vi "5.vi"(8 "error in (no error)":errorcluster) -> (0 "error out":errorcluster, 3 "Voltage":dbl)   [LabVIEW 2015]
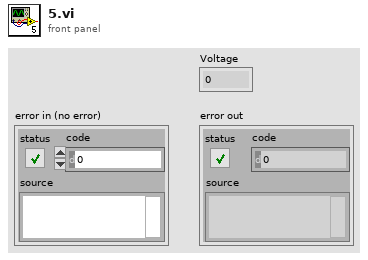
[diagram p1: front panel]
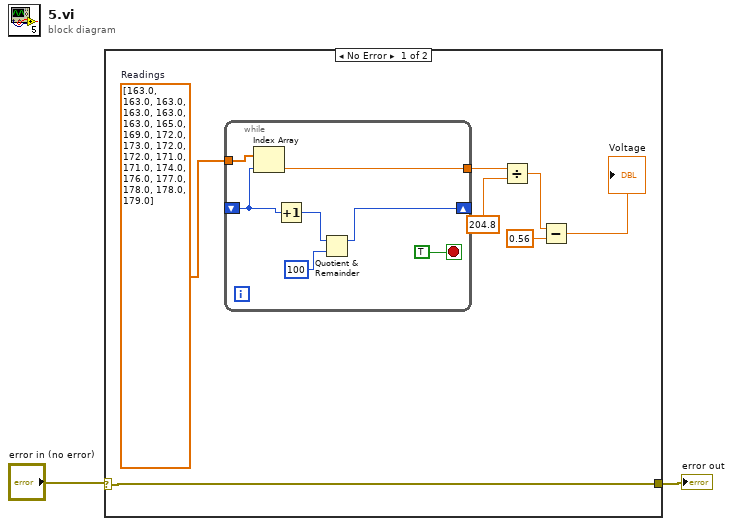
[diagram p0: block diagram]
diagram:
  n1 = case shown="No Error" "error in (no error)" {
    selector: "error in (no error)" -> [w3 w17]
    tunnel: [w3 w17] -> w1
    frame No Error {
      w4 = dbl[] [163.0, 163.0, 163.0, 163.0, 163.0, 163.0, 165.0, 169.0, 172.0, 173.0, 172.0, 172.0, 171.0, 171.0, 174.0, 176.0, 177.0, 178.0, 178.0, 179.0]  # Readings
      n2 = while {
        shift-right: [w13] -> _
        shift-left: _ -> [w12]
        tunnel: w4 -> [w11]
        tunnel: [w10] -> w7
        stop <- TRUE stop-if-true
        n3 = Index Array "Index Array"(array=w11, index=w12) -> (element=w10:dbl)
        n4 = Increment(x=w12) -> (x+1=w16:i32)
        n5 = Quotient & Remainder(x=w16, y=100) -> (x-y*floor(x/y)=w13:i32)  [unwired: 1 out]
      }
      n6 = Divide(x=w7, y=204.8) -> (x/y=w9:dbl)
      n7 = Subtract(x=w9, y=0.56) -> (x-y=→"Voltage":dbl)
    }
    frame Error {
    }
  }
  "error out" <- w1
